vi "CheckShooter.vi"(10 "Time for happy (ms)":dbl, 11 "Shooter Good?":bool) -> (3 "Good to shoot":bool)   [LabVIEW 2012]
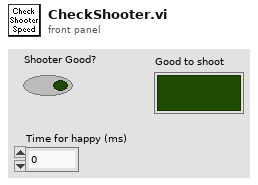
[diagram p1: front panel]
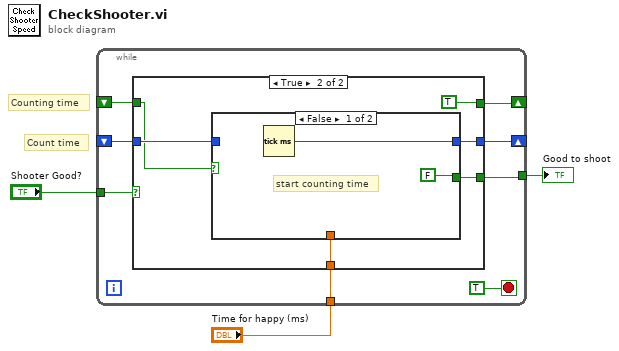
[diagram p0: block diagram]
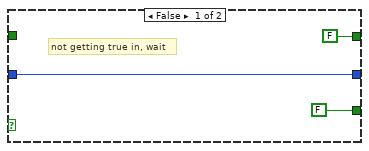
[diagram p2: hidden frame]
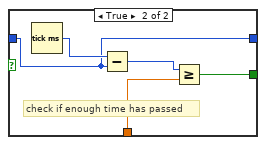
[diagram p3: hidden frame]
diagram:
  # "Count time"
  # "Counting time"
  n1 = while {
    tunnel: "Shooter Good?" -> [w11]
    tunnel: "Time for happy (ms)" -> [w10]
    tunnel: [w9] -> w1
    shift-right: [w7] -> _
    shift-left: _ -> [w8]
    shift-right: [w6] -> _
    shift-left: _ -> [w5]
    stop <- TRUE stop-if-true
    n2 = case shown="True" w11 {
      tunnel: w10 -> [_ w20]
      tunnel: [FALSE w19] -> w9
      tunnel: w8 -> [_ w16]
      tunnel: [FALSE ("Counting time") TRUE] -> w7
      tunnel: [w12 w18] -> w6
      tunnel: w5 -> [w12 w17]
      frame False {
        # "not getting true in, wait"
      }
      frame True {
        n3 = case shown="False" w16 {
          tunnel: w20 -> [_ w25]
          tunnel: [FALSE ("Counting time") w24] -> w19
          tunnel: [w21 w23] -> w18
          tunnel: w17 -> [_ w23]
          frame False {
            # "start counting time"
            n4 = Tick Count (ms)() -> (millisecond timer value=w21:u32)
          }
          frame True {
            # "check if enough time has passed"
            n5 = Tick Count (ms)() -> (millisecond timer value=w27:u32)
            n6 = Subtract(x=w27, y=w23) -> (x-y=w26:u32)
            n7 = Greater Or Equal?(x=w26, y=w25) -> (x >= y?=w24:bool)
          }
        }
      }
    }
  }
  "Good to shoot" <- w1
